vi "Update Power Supply Settings.vi"(1 "HV Out":bool, 2 "Power Supply Model":T1(ring)=enum."Keithley 24XX", 4 "Current Trip":dbl=0.005 min=0.0 max=0.005 step=1e-06 format="%.6f", 5 "Trip Mode":u16(ring) items=["Manual Trip", "Auto Trip"], 6 "Current Limit":dbl=0.0049 min=0.0 max=0.005 step=1e-06 format="%.6f", 7 "Filter Mode":u16(ring) items=["Output Filter Disabled", "Filter 1 On", "Filter 2 On"], 8 "error in":errorcluster, 9 "Voltage Level":sgl, 10 "Voltage Limit":dbl=1000.0, 11 "Power Supply Address":refnum<visa-resource-name>) -> (0 "error out":errorcluster, 3 "VISA resource name out":refnum<visa-resource-name>)   [LabVIEW 2020]
uses:
  <instrlib>/Keithley 24XX/Keithley 24XX.lvlib
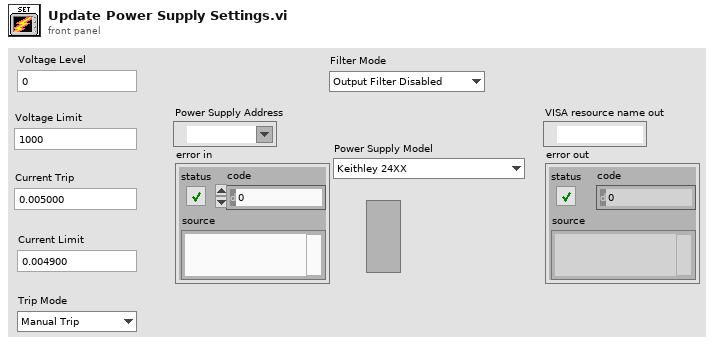
[diagram p1: front panel]
types:
  T1 = enum16{"Keithley 248", "Keithley 237", "Keithley 24XX"}
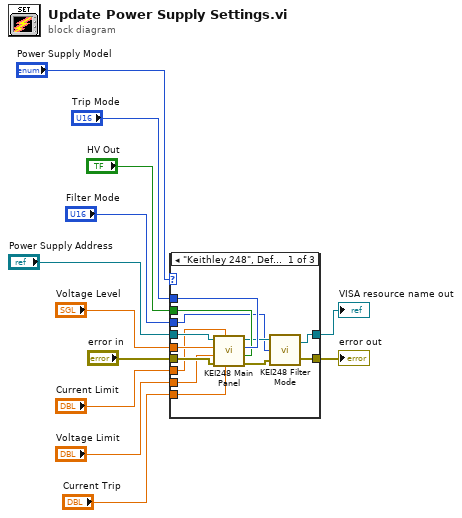
[diagram p0: block diagram]
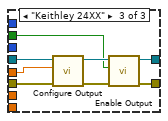
[diagram p3: hidden frame]
diagram:
  n1 = case shown="\"Keithley 248\", Default" "Power Supply Model" {
    tunnel: "Power Supply Address" -> [w25 w27 w35]
    tunnel: [w14 w26 w31] -> w8
    tunnel: "error in" -> [w24 w26 w34]
    tunnel: [w15 w27 w30] -> w9
    tunnel: "Voltage Level" -> [w23 _ w29]
    tunnel: "Voltage Limit" -> [w22 _ _]
    tunnel: "Current Limit" -> [w21 _ _]
    tunnel: "Current Trip" -> [w20 _ _]
    tunnel: "Trip Mode" -> [w19 _ _]
    tunnel: "HV Out" -> [w18 _ w28]
    tunnel: "Filter Mode" -> [w13 _ _]
    frame "Keithley 248", Default {
      n2 = call "KEI248 Main Panel"("Output Switch"=w18, "Trip Mode"=w19, "Current Trip"=w20, "Current Limit"=w21, "error in"=w24, "Voltage Limit"=w22, "Voltage Setting"=w23, "VISA resource name"=w25) -> ("error out"=w16:errorcluster, "VISA resource name out"=w17:refnum<visa-resource-name>)
      n3 = call "KEI248 Filter Mode"("error in"=w16, "Filter Mode"=w13, "VISA resource name"=w17) -> ("error out"=w14:errorcluster, "VISA resource name out"=w15:refnum<visa-resource-name>)
    }
    frame "Keithley 237" {
    }
    frame "Keithley 24XX" {
      n4 = call <instrlib>:"Configure Output.vi"("error in (no error)"=w34, "Output Level (0)"=w29, "VISA resource name"=w35) -> ("error out"=w32:errorcluster, "VISA resource name out"=w33:refnum<visa-resource-name>)  [unwired: 7 in]
      n5 = call <instrlib>:"Enable Output.vi"("error in (no error)"=w32, "Enable Output (T: Enable)"=w28, "VISA resource name"=w33) -> ("error out"=w31:errorcluster, "VISA resource name out"=w30:refnum<visa-resource-name>)  [unwired: 7 in]
    }
  }
  "VISA resource name out" <- w9
  "error out" <- w8
